vi "ZLIB Open Zip__ogtk.vi"   [LabVIEW 2013, in "ZLIB.lvlib"]
uses:
  ZLIB.lvlib
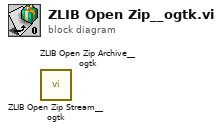
[diagram p0: block diagram]
diagram:
  n1 = call "ZLIB Open Zip Stream__ogtk.vi"() -> ()  [unwired: 5 in, 3 out]
  n2 = call "ZLIB Open Zip Archive__ogtk.vi"() -> ()  [unwired: 5 in, 3 out]
